vi "Read Position.vi"   [LabVIEW 2013, in "APU.lvclass"]
uses:
  APU/APU.lvclass
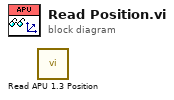
[diagram p0: block diagram]
diagram:
  n1 = call "Read APU 1.3 Position.vi"() -> ()  [unwired: 8 in, 4 out]
